vi "Colour cells.vi"() -> ()   [LabVIEW 2024]
uses:
  <vilib>/Utility/miscctls.llb/LVRowAndColumnTypeDef.ctl
  <vilib>/Utility/file.llb/Read Delimited Spreadsheet (string).vi
panel:
  out "Table":string[][](table)
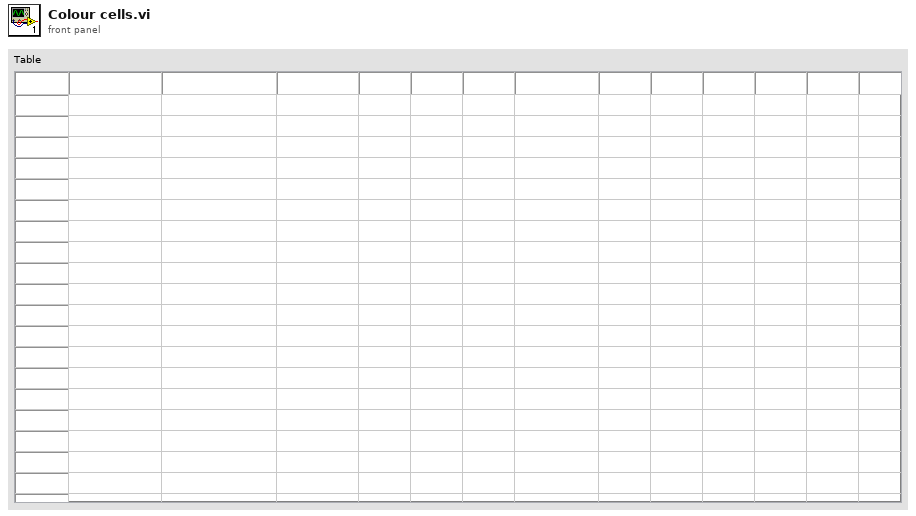
[diagram p1: front panel]
types:
  T1 = typedef "LVRowAndColumnTypeDef.ctl" = cluster{"Row":i32, "Column":i32}
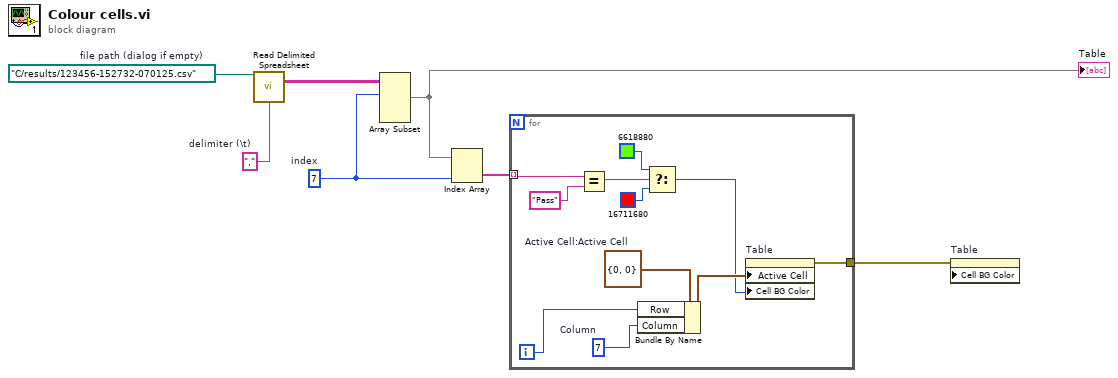
[diagram p0: block diagram]
diagram:
  w2 = 7  # index
  w6 = ","  # delimiter (\t)
  w7 = path "C:/results/123456-152732-070125.csv"  # file path (dialog if empty)
  n1 = call-poly <vilib>:"Read Delimited Spreadsheet.vi"("file path (dialog if empty)"=w7, "delimiter (\\t)"=w6) -> ("all rows"=w5:string[][])  [unwired: 8 in, 5 out]
  n2 = Array Subset(array=w5, index (row)=w2) -> (w4:string[][])  [unwired: 3 in]
  "Table" <- w4
  n3 = Index Array(array=w4, index (col)=w2) -> (element=w3:string[])  [unwired: 1 in]
  n4 = for {
    tunnel: w3 -> [w18] mode=indexing
    tunnel: [w8] -> w1
    i -> [w12]
    w11 = 7  # Column
    w13 = T1 {"Row"=0, "Column"=0}  # Active Cell:Active Cell
    n5 = Equal?(x=w18, y="Pass") -> (x = y?=w16:bool)
    n6 = Bundle By Name(cluster=w13, "Row"=w12, "Column"=w11) -> (w10:T1)
    n7 = Select(t=u32 6618880, s=w16, f=u32 16711680) -> (s? t:f=w9:u32)
    n8 = property on="Table" class="Tbl (strict)"("Active Cell"=w10, "Cell BG Color"=w9) -> (error out=w8:errorcluster)  [unwired: 2 in, 1 out]
  }
  n9 = property on="Table" class="Tbl (strict)" props=["Cell BG Color"](error in=w1) -> ()  [unwired: 2 in, 2 out]
